vi "BuildNyquist.vi"(9 "subset":cluster{"Min":dbl, "Max":dbl}={"Min"=0.0, "Max"=100000.0}, 11 "Complex FRF":cluster{"t0":dbl, "dt":dbl, "Y":cdb[]}) -> (0 "Phase":cluster{"t0":dbl, "dt":dbl, "Y":dbl[]}(graph), 1 "plots out":refnum<class "Base Datatype.lvclass">[](array[class]), 2 "Nyquist Plot":cluster{dbl[], dbl[]}(graph), 3 "Energy":cluster{"x0":dbl, "df":dbl, dbl[]}[](graph))   [LabVIEW 2022 SP3]
uses:
  <vilib>/Native 3D Graph/xcontrol/3DPC_SurfacePlot.xctl
  <vilib>/Native 3D Graph/classes/Base Datatype.lvclass
panel:
  out "Array":T1(array[cluster]) {"r" format="%.6f"}
  out "3D Nyquist":refnum<class "Base Datatype.lvclass">[](xcontrol)
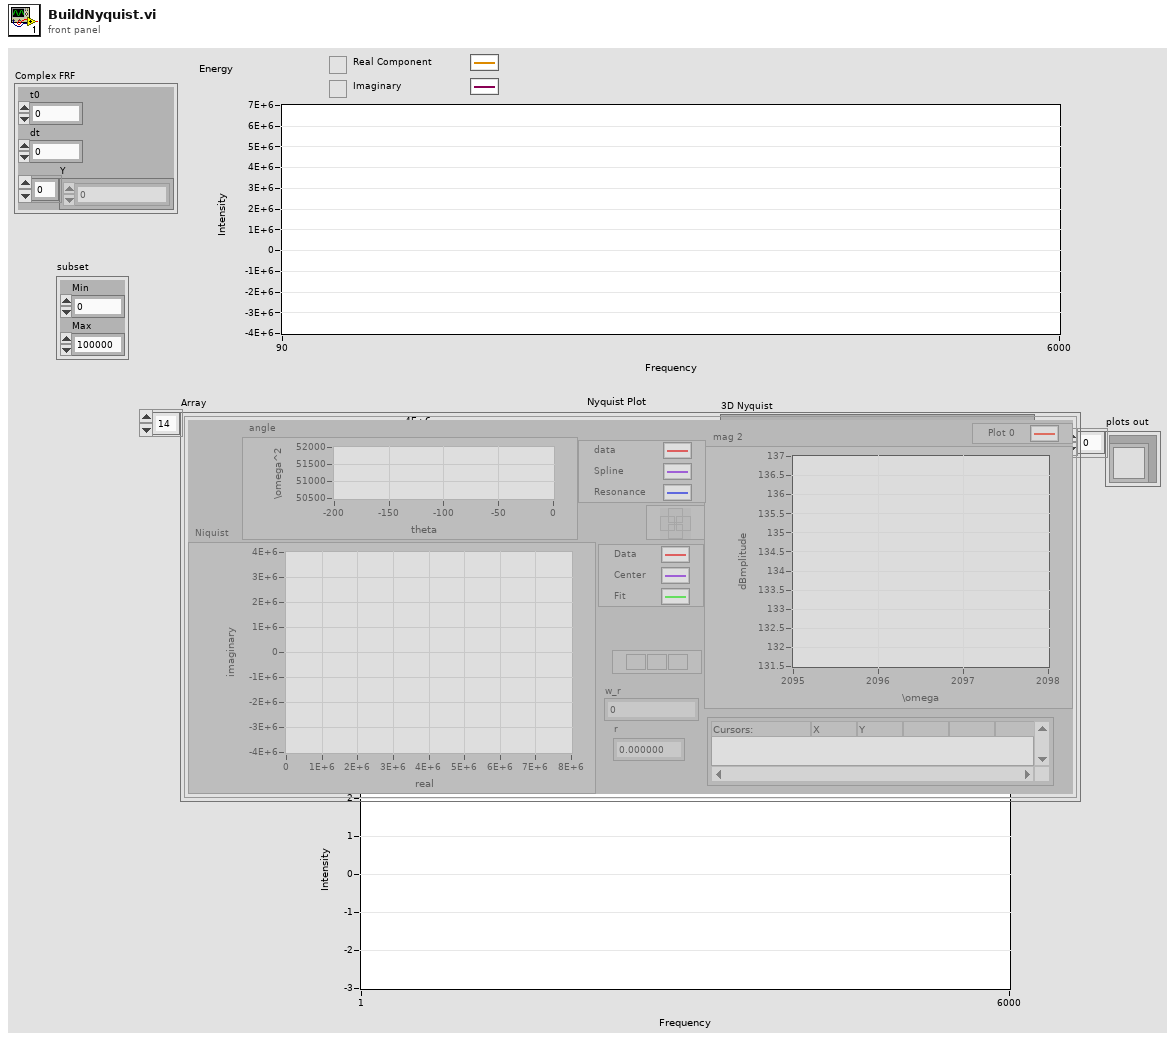
[diagram p1: front panel]
types:
  T1 = cluster{"angle":cluster{dbl[], "yi":dbl[]}[], "Niquist":cluster{dbl[], dbl[]}[], "mag 2":cluster{dbl[], dbl[]}, "w_r":dbl, "r":dbl}[]
  T2 = cluster{"angle":cluster{dbl[], "yi":dbl[]}[], "Niquist":cluster{dbl[], dbl[]}[], "mag 2":cluster{dbl[], dbl[]}, "w_r":dbl, "r":dbl}
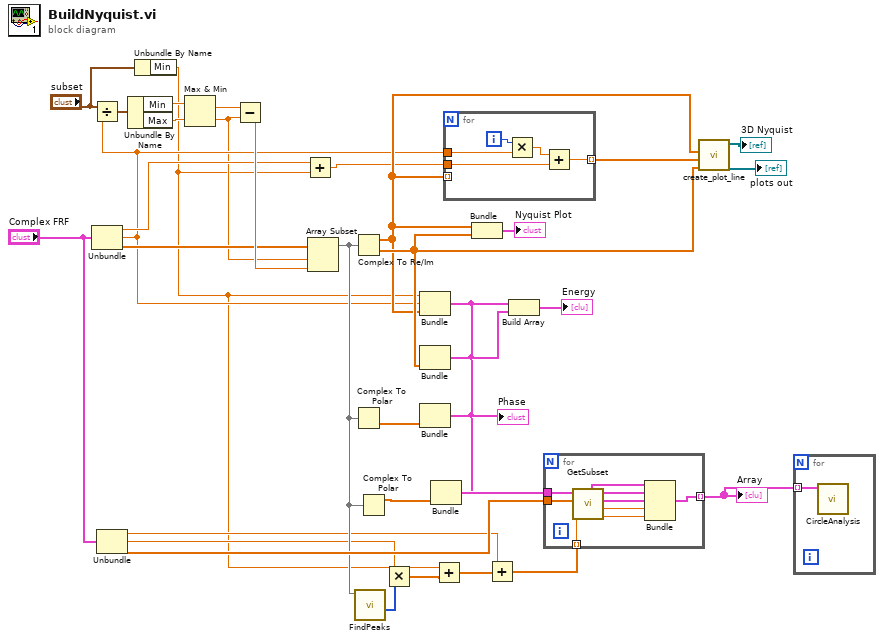
[diagram p0: block diagram]
diagram:
  n1 = Unbundle("Complex FRF") -> ("t0"=w21:dbl, "dt"=w7:dbl, "Y"=w22:cdb[])
  n2 = Divide(x="subset", y=w7) -> (x/y=w4:cluster{"Min":dbl, "Max":dbl})
  n3 = Unbundle("Complex FRF") -> ("t0"=w13:dbl, "dt"=w14:dbl, "Y"=w20:cdb[])
  n4 = Unbundle By Name(w4) -> ("Min"=w5:dbl, "Max"=w25:dbl)
  n5 = Unbundle By Name("subset") -> ("Min"=w2:dbl)
  n6 = Max & Min(x=w5, y=w25) -> (max(x,y)=w24:dbl, min(x,y)=w6:dbl)
  n7 = Subtract(x=w24, y=w6) -> (x-y=w23:dbl)
  n8 = Add(x=w21, y=w2) -> (x+y=w11:dbl)
  n9 = Array Subset(array=w22, index=w6, length=w23) -> (w15:cdb[])
  n10 = Complex To Re/Im(x + iy=w15) -> (x=w27:dbl[], y=w28:dbl[])
  n11 = Complex To Polar(r * e^(i*theta)=w15) -> (theta=w33:dbl[])  [unwired: 1 out]
  n12 = call "FindPeaks.vi"("subarray"=w15) -> ("indicies"=w10:i32[])  [unwired: 10 in]
  n13 = Complex To Polar(r * e^(i*theta)=w15) -> (r=w16:dbl[])  [unwired: 1 out]
  n14 = Multiply(x=w14, y=w10) -> (x*y=w9:dbl[])
  n15 = Bundle("Min"=w2, "dt"=w7, w27) -> (w17:cluster{"Min":dbl, "dt":dbl, dbl[]})  [unwired: 1 in]
  n16 = Bundle(cluster=w17, w28) -> (w31:cluster{"Min":dbl, "dt":dbl, dbl[]})  [unwired: 2 in]
  n17 = Bundle(cluster=w17, w33) -> (→"Phase":cluster{"Min":dbl, "dt":dbl, dbl[]})  [unwired: 2 in]
  n18 = Bundle(cluster=w17, w16) -> (w19:cluster{"Min":dbl, "dt":dbl, dbl[]})  [unwired: 2 in]
  n19 = Add(x=w2, y=w9) -> (x+y=w8:dbl[])
  n20 = for {
    tunnel: w27 -> [_] mode=indexing
    tunnel: w7 -> [w38]
    tunnel: w11 -> [w36]
    tunnel: [w35] -> w29 mode=indexing
    i -> [w39]
    n21 = Multiply(x=w39, y=w38) -> (x*y=w37:dbl)
    n22 = Add(x=w37, y=w36) -> (x+y=w35:dbl)
  }
  n23 = Bundle(w27, w28) -> (→"Nyquist Plot":cluster{dbl[], dbl[]})  [unwired: 1 in]
  n24 = Add(x=w13, y=w8) -> (x+y=w12:dbl[])
  n25 = Build Array(w17, w31) -> (→"Energy":cluster{"Min":dbl, "dt":dbl, dbl[]}[])
  n26 = for {
    tunnel: w20 -> [w48]
    tunnel: w19 -> [w47]
    tunnel: w12 -> [w46] mode=indexing
    tunnel: [w45] -> w1 mode=indexing
    n27 = call "GetSubset.vi"("omega"=w46, "FFT"=w48, "mag"=w47) -> ("r"=w41:dbl, "w_r"=w42:dbl, "mag 2"=w43:cluster{dbl[], dbl[]}, "Niquist"=w44:cluster{dbl[], dbl[]}[], "angle"=w40:cluster{dbl[], "yi":dbl[]}[])  [unwired: 4 in]
    n28 = Bundle("angle"=w40, "Niquist"=w44, "mag 2"=w43, "w_r"=w42, "r"=w41) -> (w45:T2)  [unwired: 1 in]
  }
  "Array" <- w1
  n29 = call <vilib>:"create_plot_line.vi"("z vector"=w28, "y vector"=w29, "x vector"=w27) -> ("plots out"=→"3D Nyquist" →"plots out":refnum<class "Base Datatype.lvclass">[])  [unwired: 2 in, 6 out]
  n30 = for {
    tunnel: w1 -> [w49] mode=indexing
    n31 = call "CircleAnalysis.vi"("Cluster"=w49) -> ()  [unwired: 11 in]
  }
